vi "ex_Disable.vi"(1 "Disable?":bool) -> (0 "Disabled value":u8)   [LabVIEW 2017]
doc: "Returns a value of 2 if Disable? is TRUE, otherwise returns 0."
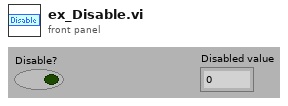
[diagram p1: front panel]
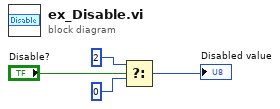
[diagram p0: block diagram]
diagram:
  n1 = Select(t=u8 2 ("f"), s="Disable?", f=u8 0 ("t")) -> (s? t:f=→"Disabled value":u8)
